vi "VectorDisplay.vi"(7 "Ref for Sizing":refnum<vi>, 8 "Colormap.Value Max":dbl, 11 "Array":csg[][](array[numeric])) -> (3 "Vector Plot":picture)   [LabVIEW 2022 SP3]
uses:
  <vilib>/Heliosphere Research LLC/Advanced Plotting Toolkit/typedefs/PlotColor.ctl
  <vilib>/Heliosphere Research LLC/Advanced Plotting Toolkit/api_core/NewPlotProperties.ctl
  <vilib>/Heliosphere Research LLC/Advanced Plotting Toolkit/properties/Colormap_Map.ctl
  <vilib>/Heliosphere Research LLC/Advanced Plotting Toolkit/properties/Colormap_Scaling.ctl
  <vilib>/Heliosphere Research LLC/Advanced Plotting Toolkit/properties/Colormap.ctl
  <vilib>/Heliosphere Research LLC/Advanced Plotting Toolkit/properties/Display.ctl
  <vilib>/Heliosphere Research LLC/Advanced Plotting Toolkit/api_plotting/VectorFieldProperties.ctl
panel:
  in  "Arrow Colors":T1(ring)=enum."X Vector Component"
  # "Vector Field"
  # "This VI demonstrates the simplest way to visualize a vector\nfield: by plotting a field of arrows.\n\nA pair of 2D arrays are provided, one which gives the X\ncomponent at every point, and one which give the Y\ncomponent at every point.  The Toolkit then paints an arrow\nat each point of the appropriate size and direction.\n\nBy default, all the arrows will be colored black.  But if you\nsupply another 2D array to the Colormap Values input, its\nvalues will be used to color the arrows.\n\nThis demo shows the magnetic field around a wire of\nfinite size.  You can choose whether to color the arrows\naccording to the X or Y components, or the overall\nmagnitude of the vector at each point."
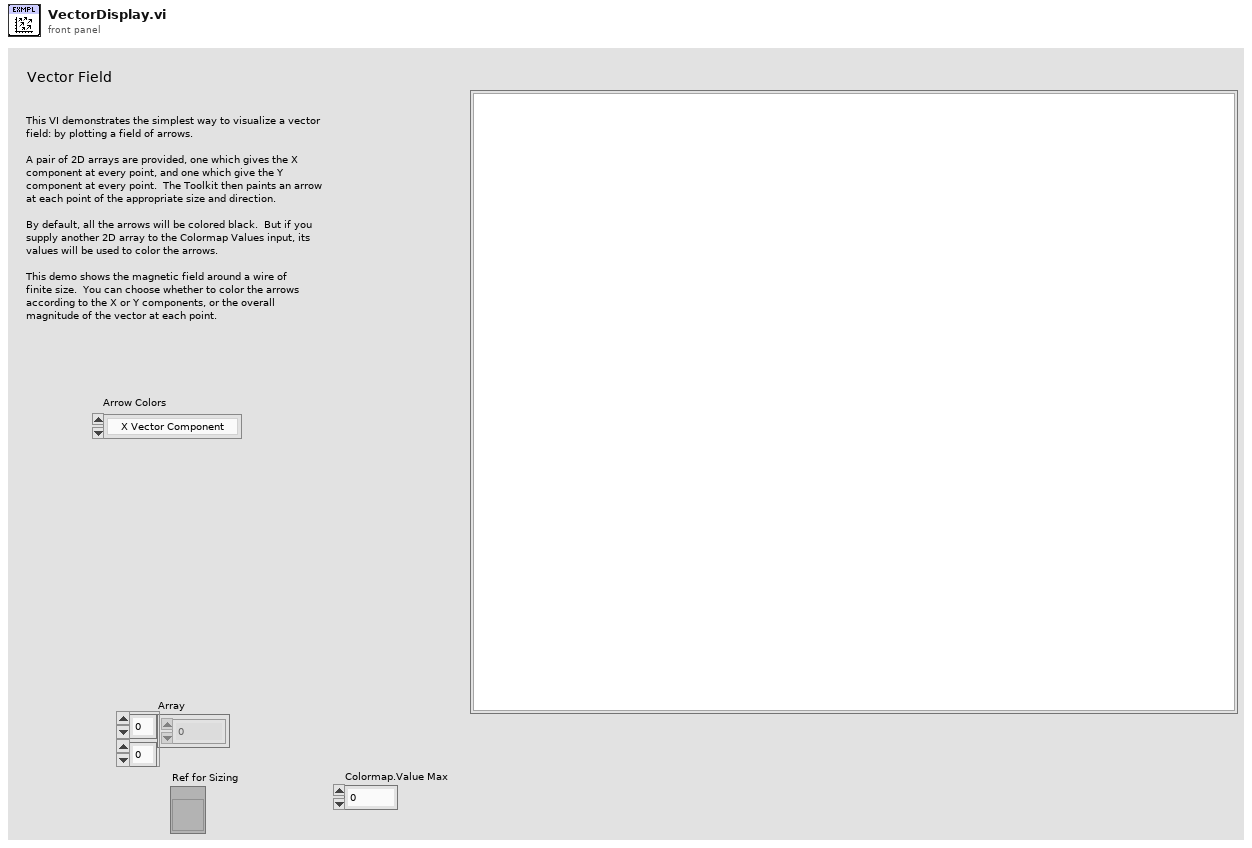
[diagram p1: front panel]
types:
  T1 = enum16{"Vector Magnitude", "X Vector Component", "Y Vector Component", "Plain Black"}
  T2 = typedef "Advanced Plotting Toolkit.lvlib/Colormap_Map.ctl" = enum16{"Automatic", "Rainbow", "Hot and Cold", "White-Black", "White-Blue", "White-Green", "White-Red", "Fire", "Water", "Earth", "Air", "Pastel", "Banded", "Stepped"}
  T3 = typedef "Advanced Plotting Toolkit.lvlib/VectorFieldProperties.ctl" = cluster{"Color":T4, "Arrow Scale":dbl, "Colormap":T5, "Display":T7}
  T4 = typedef "Advanced Plotting Toolkit.lvlib/PlotColor.ctl" = u32
  T5 = typedef "Advanced Plotting Toolkit.lvlib/Colormap.ctl" = cluster{"Map":T2, "Value Min":dbl, "Value Max":dbl, "Scaling":T6, "Reverse":bool}
  T6 = typedef "Advanced Plotting Toolkit.lvlib/Colormap_Scaling.ctl" = enum16{"Default"}
  T7 = typedef "Advanced Plotting Toolkit.lvlib/Display.ctl" = cluster{"Alpha":dbl, "Z Order":dbl}
  T8 = typedef "Advanced Plotting Toolkit.lvlib/NewPlotProperties.ctl" = cluster{"Background Color":T4, "Axis Background":T4, "Left Margin":dbl, "Right Margin":dbl, "Bottom Margin":dbl, "Top Margin":dbl, "Aspect Ratio":dbl}
  T9 = typedef "Advanced Plotting Toolkit.lvlib/PlotID.ctl" = i32
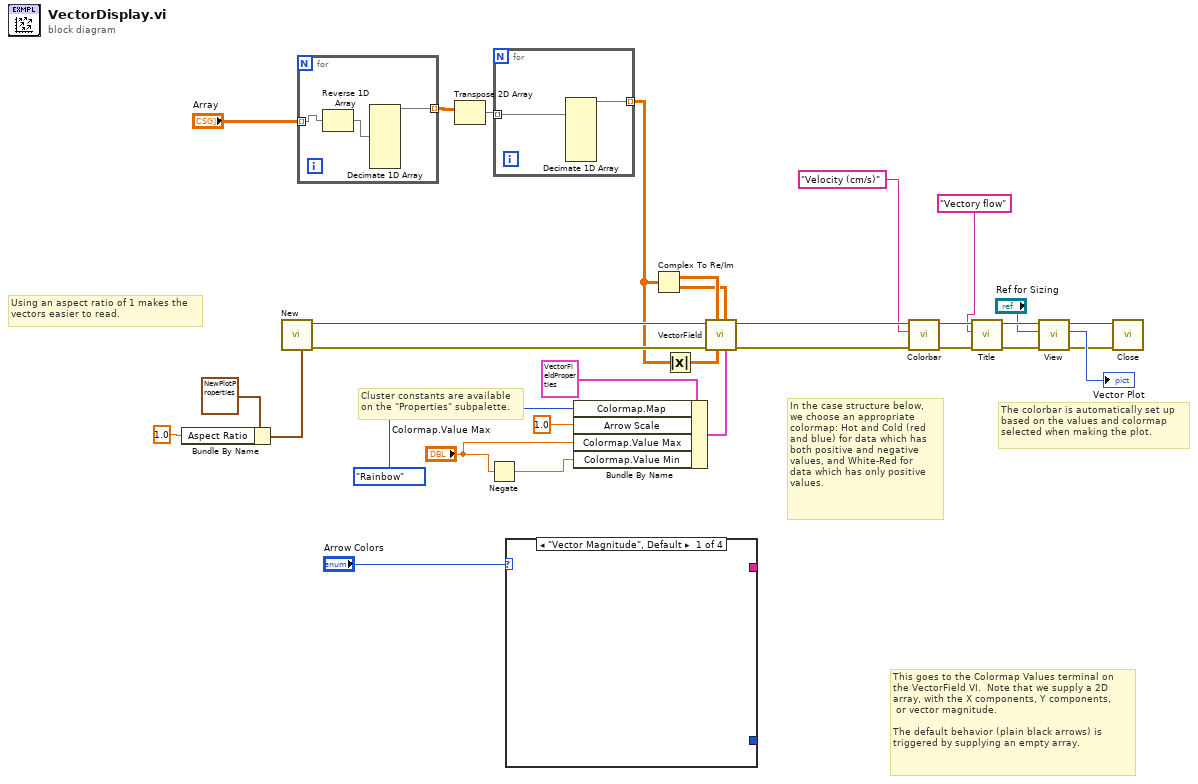
[diagram p0: block diagram]
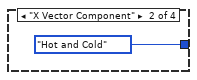
[diagram p2: hidden frame]
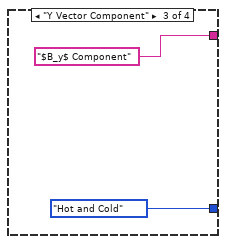
[diagram p3: hidden frame]
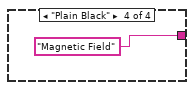
[diagram p4: hidden frame]
diagram:
  # "Cluster constants are available\non the \"Properties\" subpalette."
  # "In the case structure below,\nwe choose an appropriate\ncolormap: Hot and Cold (red\nand blue) for data which has\nboth positive and negative\nvalues, and White-Red for\ndata which has only positive\nvalues."
  # "The colorbar is automatically set up\nbased on the values and colormap \nselected when making the plot."
  # "This goes to the Colormap Values terminal on\nthe VectorField VI.  Note that we supply a 2D\narray, with the X components, Y components,\n or vector magnitude.\n\nThe default behavior (plain black arrows) is\ntriggered by supplying an empty array."
  # "Using an aspect ratio of 1 makes the\nvectors easier to read."
  n1 = Bundle By Name(cluster=T8 {"Background Color"=2147483647, "Axis Background"=2147483647, "Left Margin"=nan, "Right Margin"=nan, "Bottom Margin"=nan, "Top Margin"=nan, "Aspect Ratio"=nan} ("New Plot Properties"), "Aspect Ratio"=1.0) -> (w24:T8)
  n2 = call <vilib>:"New.vi"("Properties"=w24) -> ("error out"=w23:errorcluster, "Plot ID"=w29:T9)  [unwired: 9 in]
  n3 = for {
    tunnel: "Array" -> [w33] mode=indexing
    tunnel: [w34] -> w13 mode=indexing
    n4 = Reverse 1D Array(array=w33) -> (reversed array=w32:csg[])
    n5 = Decimate 1D Array(w32) -> (w34:csg[])  [unwired: 7 out]
  }
  n6 = Transpose 2D Array(2D array=w13) -> (transposed array=w12:csg[][])
  n7 = Negate(x="Colormap.Value Max") -> (-x=w1:dbl)
  n8 = for {
    tunnel: w12 -> [w36] mode=indexing
    tunnel: [w35] -> w7 mode=indexing
    n9 = Decimate 1D Array(w36) -> (w35:csg[])  [unwired: 7 out]
  }
  n10 = case shown="\"Vector Magnitude\", Default" "Arrow Colors" {
    tunnel: [_ Colormap_Map."Hot and Cold" ("Colormap.Map") Colormap_Map."Hot and Cold" ("Colormap.Map") _] -> _
    tunnel: [_ _ "$B_y$ Component" "Magnetic Field"] -> _
    frame "Vector Magnitude", Default {
    }
    frame "X Vector Component" {
    }
    frame "Y Vector Component" {
    }
    frame "Plain Black" {
    }
  }
  n11 = Bundle By Name(cluster=T3 {"Color"=2147483647, "Arrow Scale"=nan, "Colormap"={"Map"=enum."Automatic", "Value Min"=nan, "Value Max"=nan, "Scaling"=enum."Default", "Reverse"=FALSE}, "Display"={"Alpha"=nan, "Z Order"=nan}} ("Vector Field Properties"), "Colormap.Map"=Colormap_Map."Rainbow", "Arrow Scale"=1.0, "Colormap.Value Max"="Colormap.Value Max", "Colormap.Value Min"=w1) -> (w20:T3)
  n12 = Complex To Re/Im(x + iy=w7) -> (x=w9:sgl[][], y=w8:sgl[][])
  n13 = Absolute Value(x=w7) -> (abs(x)=w6:sgl[][])
  n14 = call <vilib>:"VectorField.vi"("Properties"=w20, "Y Vector Component"=w8, "Colormap Values"=w6, "X Vector Component"=w9, "error in (no error)"=w23, "Plot ID"=w29) -> ("error out"=w22:errorcluster, "Plot ID Out"=w27:T9)  [unwired: 4 in]
  n15 = call <vilib>:"Colorbar.vi"("error in (no error)"=w22, "Label"="Velocity (cm/s)", "Plot ID"=w27) -> ("error out"=w18:errorcluster, "Plot ID Out"=w19:T9)  [unwired: 7 in]
  n16 = call <vilib>:"Title.vi"("error in (no error)"=w18, "Title"="Vectory flow", "Plot ID"=w19) -> ("error out"=w16:errorcluster, "Plot ID out"=w17:T9)  [unwired: 7 in]
  n17 = call <vilib>:"View.vi"("error in (no error)"=w16, "Ref for Sizing"="Ref for Sizing", "Plot ID"=w17) -> ("error out"=w14:errorcluster, "Picture"=→"Vector Plot":picture, "Plot ID Out"=w30:T9)  [unwired: 6 in]
  n18 = call <vilib>:"Close.vi"("error in (no error)"=w14, "Plot ID"=w30) -> ()  [unwired: 9 in, 1 out]
